vi "read 12V monitor from Z SDI-12 address.vi"(8 "error in (no error)":errorcluster, 11 "List of Com Ports Present in System":refnum<visa-resource-name>[](array[refnum])) -> (0 "error out":errorcluster, 1 "12V monitor":dbl, 2 "H-4191 Adapter found":bool, 3 "List of Com Ports Present in System 2":refnum<visa-resource-name>[](array[refnum]))   [LabVIEW 2016]
uses:
  SDI-12/SDI-12.lvlib
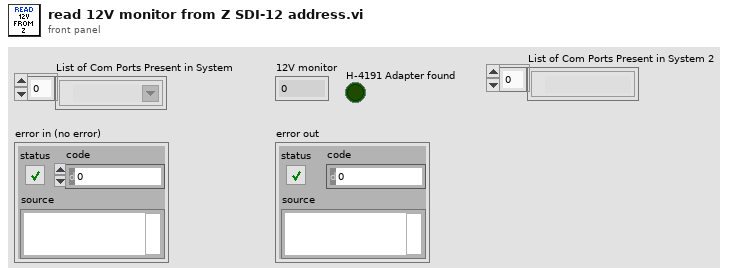
[diagram p1: front panel]
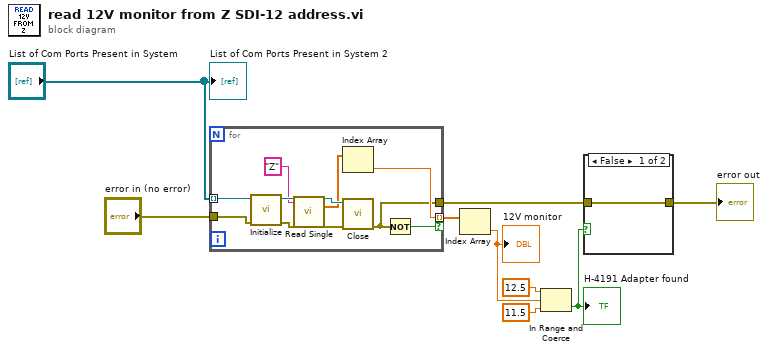
[diagram p0: block diagram]
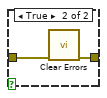
[diagram p2: hidden frame]
diagram:
  n1 = for {
    tunnel: "List of Com Ports Present in System" -> [w20] mode=indexing
    tunnel: "error in (no error)" -> [w19]
    tunnel: [w11] -> w8
    tunnel: [w12] -> w3 mode=indexing if=w10
    n2 = call "Initialize.vi"("Error In (No Error)"=w19, "RS232 Port In"=w20) -> ("Error Out"=w17:errorcluster, "RS232 Port Out"=w18:refnum<visa-resource-name>)  [unwired: 8 in]
    n3 = call "Read Single.vi"("RS232 Port In"=w18, "Sensor Address In"="Z", "Error In (No Error)"=w17) -> ("RS232 Port Out"=w15:refnum<visa-resource-name>, "Measurements Out"=w13:dbl[], "Error Out"=w16:errorcluster)  [unwired: 17 in, 5 out]
    n4 = Index Array(array=w13) -> (element=w12:dbl)  [unwired: 1 in]
    n5 = call "Close.vi"("Error In (No Error)"=w16, "RS232 Port In"=w15) -> ("Error Out"=w11:errorcluster)  [unwired: 9 in]
    n6 = Not(x=w11) -> (.not. x?=w10:bool)
  }
  n7 = Index Array(array=w3) -> (element=w4:dbl)  [unwired: 1 in]
  "12V monitor" <- w4
  n8 = In Range and Coerce(upper limit=12.5, x=w4, lower limit=11.5) -> (In Range?=w7:bool)  [unwired: 1 out]
  "H-4191 Adapter found" <- w7
  n9 = case shown="False" w7 {
    tunnel: w8 -> [w21 w23]
    tunnel: [w21 w22] -> w9
    frame False {
    }
    frame True {
      n10 = call <vilib>:"Clear Errors.vi"("error in (no error)"=w23) -> ("error out"=w22:errorcluster)  [unwired: 5 in, 1 out]
    }
  }
  "error out" <- w9
  "List of Com Ports Present in System 2" <- "List of Com Ports Present in System"
